vi "NoServicesRegistered_InvalidRegisterRequests_Error.vi"() -> (6 "Pass":bool, 15 "error out":errorcluster)   [LabVIEW 2020]
uses:
  Discovery_client/RPC Messages/ni_measurements_discovery_v1_RegisterServiceRequest.ctl
  Discovery_client/RPC Messages/ni_measurements_discovery_v1_ServiceDescriptor.ctl
  Discovery_client/RPC Messages/ni_measurements_discovery_v1_ServiceLocation.ctl
  <vilib>/ErrorRing/Error Ring.xnode
  Discovery_client/Discovery_client.lvlib
panel:
  out "Empty insecure_port fails (as expected)?":bool
  out "Empty display_name fails (as expected)?":bool
  out "Empty location fails (as expected)?":bool
  out "Empty service_class fails (as expected)?":bool
  out "Empty provided_interfaces fails (as expected)?":bool
  # "Test assumes discovery service has already been started."
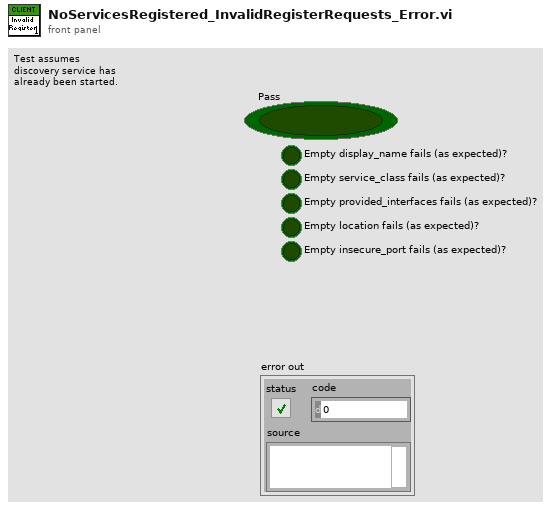
[diagram p1: front panel]
types:
  T1 = typedef "Discovery_client.lvlib/ni_measurements_discovery_v1_RegisterServiceRequest.ctl" = cluster{"service_description":T2, "location":T3}
  T2 = typedef "Discovery_client.lvlib/ni_measurements_discovery_v1_ServiceDescriptor.ctl" = cluster{"display_name":string, "description_url":string, "provided_interfaces":string[], "service_class":string, "attributes":string[]}
  T3 = typedef "Discovery_client.lvlib/ni_measurements_discovery_v1_ServiceLocation.ctl" = cluster{"location":string, "insecure_port":string, "ssl_authenticated_port":string}
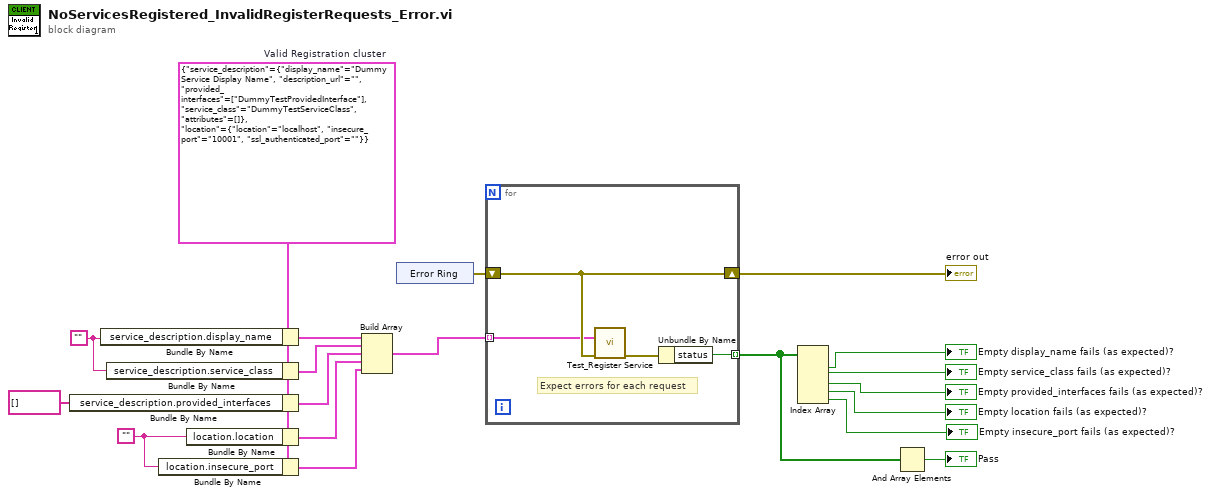
[diagram p0: block diagram]
diagram:
  w3 = ""
  w8 = ""
  w2 = T1 {"service_description"={"display_name"="Dummy Service Display Name", "description_url"="", "provided_interfaces"=["DummyTestProvidedInterface"], "service_class"="DummyTestServiceClass", "attributes"=[]}, "location"={"location"="localhost", "insecure_port"="10001", "ssl_authenticated_port"=""}}  # Valid Registration cluster
  n1 = Bundle By Name(cluster=w2, "service_description.provided_interfaces"=string[] []) -> (w6:T1)
  n2 = Bundle By Name(cluster=w2, "service_description.display_name"=w8) -> (w9:T1)
  n3 = Bundle By Name(cluster=w2, "service_description.service_class"=w8) -> (w7:T1)
  n4 = Bundle By Name(cluster=w2, "location.insecure_port"=w3) -> (w1:T1)
  n5 = Bundle By Name(cluster=w2, "location.location"=w3) -> (w4:T1)
  n6 = Build Array(w9, w7, w6, w4, w1) -> (w10:T1[])
  n7 = xnode "Error Ring"() -> ("error out"=w12:errorcluster)
  n8 = for {
    tunnel: [w23] -> w14 mode=indexing
    tunnel: w10 -> [w21] mode=indexing
    shift-right: [w22] -> w11
    shift-left: w12 -> [w22]
    # "Expect errors for each request"
    n9 = call "Test_Register Service.vi"("Request Data"=w21, "error in (no error)"=w22) -> ("error out"=w20:errorcluster)  [unwired: 12 in, 1 out]
    n10 = Unbundle By Name(w20) -> ("status"=w23:bool)
  }
  "error out" <- w11
  n11 = Index Array(array=w14) -> (element #1=→"Empty display_name fails (as expected)?":bool, element #2=→"Empty service_class fails (as expected)?":bool, element #3=→"Empty provided_interfaces fails (as expected)?":bool, element #4=→"Empty location fails (as expected)?":bool, element #5=→"Empty insecure_port fails (as expected)?":bool)  [unwired: 5 in]
  n12 = And Array Elements(Boolean array=w14) -> (logical AND=→"Pass":bool)
